vi "Arrange VIWin - Get Window INI tokens.vi"(0 "window type":T5, 11 "error in":errorcluster) -> (4 "Window INI tokens":T4, 15 "error out":errorcluster)   [LabVIEW 2012, in "Arrange VI Window.lvlib"]
uses:
  Arrange VI Window.lvlib
  Arrange VIWin - Window Type.ctl
  <vilib>/Utility/miscctls.llb/LVRectTypeDef.ctl
  Arrange VIWin - Min Window Dimensions.ctl
  Arrange VIWin - Window Gaps.ctl
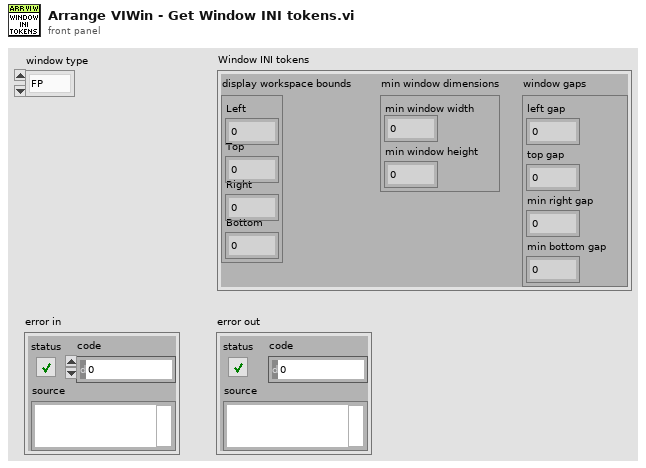
[diagram p1: front panel]
types:
  T1 = typedef "LVRectTypeDef.ctl" = cluster{"Left":i16, "Top":i16, "Right":i16, "Bottom":i16}
  T2 = typedef "Arrange VI Window.lvlib/Arrange VIWin - Min Window Dimensions.ctl" = cluster{"min window width":i16, "min window height":i16}
  T3 = typedef "Arrange VI Window.lvlib/Arrange VIWin - Window Gaps.ctl" = cluster{"left gap":i16, "top gap":i16, "min right gap":i16, "min bottom gap":i16}
  T4 = cluster{"display workspace bounds":T1, "min window dimensions":T2, "window gaps":T3}
  T5 = typedef "Arrange VI Window.lvlib/Arrange VIWin - Window Type.ctl" = enum16{"FP", "BD"}
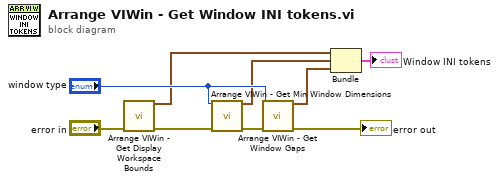
[diagram p0: block diagram]
diagram:
  n1 = call "Arrange VIWin - Get Display Workspace Bounds.vi"("error in"="error in") -> ("display workspace bounds"=w4:T1, "error out"=w8:errorcluster)  [unwired: 13 in]
  n2 = call "Arrange VIWin - Get Min Window Dimensions.vi"("window type"="window type", "error in"=w8) -> ("min window dimensions"=w3:T2, "error out"=w7:errorcluster)  [unwired: 12 in]
  n3 = call "Arrange VIWin - Get Window Gaps.vi"("window type"="window type", "error in"=w7) -> ("window gaps"=w2:T3, "error out"=→"error out":errorcluster)  [unwired: 12 in]
  n4 = Bundle("display workspace bounds"=w4, "min window dimensions"=w3, "window gaps"=w2) -> (→"Window INI tokens":T4)  [unwired: 1 in]
